vi "Read configuration.vi"(8 "error in":errorcluster, 11 "Modbus Slave editor node in":refnum<class "Modbus Module editor node.lvclass">) -> (0 "error out":errorcluster, 2 "configuration":refnum<class "NISE_CEF_serializable configuration.lvclass">, 3 "Modbus Slave editor node out":refnum<class "Modbus Module editor node.lvclass">)   [LabVIEW 2015, in "Modbus Module editor node.lvclass"]
doc: "Platypus Framework 1.0.1.65\nNI Systems Engineering - National Instruments"
uses:
  Modbus Module editor node.lvclass
  <vilib>/NI/Configuration Framework/serializable configuration/NISE_CEF_serializable configuration.lvclass
  Modbus Module editor node.lvclass/Modbus Module editor node.ctl
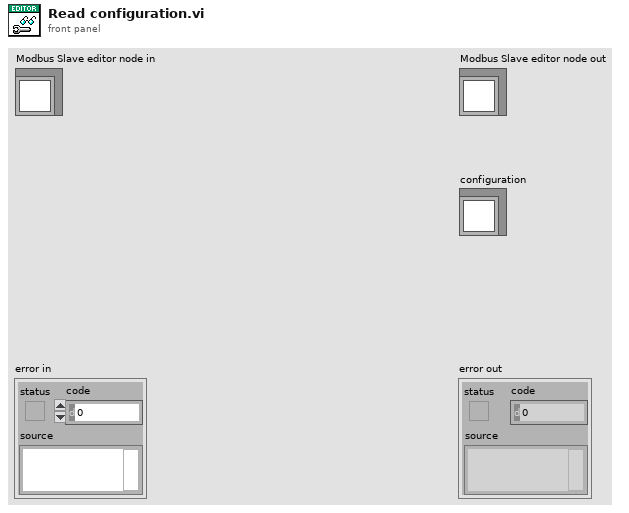
[diagram p1: front panel]
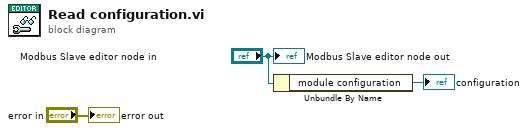
[diagram p0: block diagram]
diagram:
  n1 = Unbundle By Name("Modbus Slave editor node in") -> ("module configuration"=→"configuration":refnum<class "Modbus Module configuration.lvclass">)
  "error out" <- "error in"
  "Modbus Slave editor node out" <- "Modbus Slave editor node in"
